vi "PICInit.vi"(2 "Error In":errorcluster, 3 "Enum":enum32{"9600", "115200"}(ring), 4 "VISA resource name":refnum<visa-resource-name>) -> (0 "error out":errorcluster, 1 "VISA resource name out":refnum<visa-resource-name>)   [LabVIEW 2012]
uses:
  <vilib>/Instr/_visa.llb/VISA Find Search Mode.ctl
  <vilib>/Instr/_visa.llb/VISA Configure Serial Port (Instr).vi
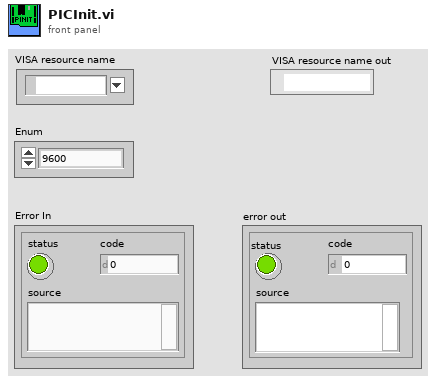
[diagram p1: front panel]
types:
  T1 = typedef "VISA Find Search Mode.ctl" = u32
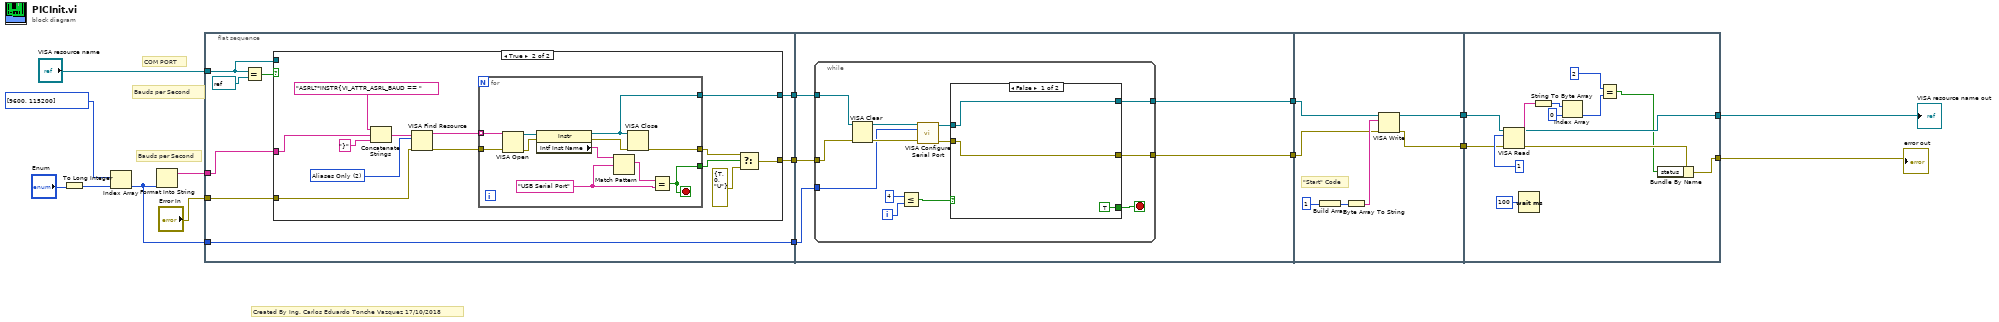
[diagram p0: block diagram]
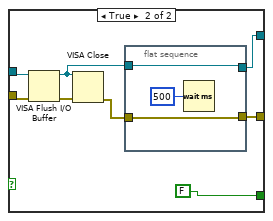
[diagram p3: hidden frame]
diagram:
  # "Created By Ing. Carlos Eduardo Tonche Vazquez 17/10/2018"
  # "COM PORT"
  # "Bauds per Second"
  # "Bauds per Second"
  n1 = To Long Integer(number="Enum") -> (32bit integer=w14:i32)
  n2 = Index Array(array=u32[] [9600, 115200], index=w14) -> (element=w11:u32)
  n3 = Format Into String(w11) -> (resulting string=w13:string)  [unwired: 3 in, 1 out]
  n4 = flat-sequence {
    tunnel: w13 -> [w22]
    tunnel: "VISA resource name" -> [w18]
    tunnel: w11 -> [w17]
    tunnel: "Error In" -> [w21]
    tunnel: [w20] -> w9
    tunnel: [w19] -> w8
    tunnel: [w17] -> w7
    tunnel: w9 -> [w55]
    tunnel: w8 -> [w54]
    tunnel: w7 -> [w53]
    tunnel: [w52] -> w6
    tunnel: [w51] -> w5
    tunnel: w6 -> [w86]
    tunnel: w5 -> [w85]
    tunnel: [w84] -> w2
    tunnel: [w83] -> w1
    tunnel: [w93] -> w3
    tunnel: [w92] -> w4
    tunnel: w2 -> [w95]
    tunnel: w1 -> [w94]
    frame #0 {
      n5 = Equal?(x=w18, y=refnum<visa-resource-name> refnum) -> (x = y?=w23:bool)
      n6 = case shown="True" w23 {
        tunnel: w22 -> [_ w37]
        tunnel: w21 -> [w25 w34]
        tunnel: [w25 w28] -> w20
        tunnel: [w26 w27] -> w19
        tunnel: w18 -> [w26 _]
        frame False {
        }
        frame True {
          w35 = T1 2 items=["Canonical Names Only"=0, "Aliases Only"=2, "Include Matching Aliases"=3, "Include All Aliases"=4] ("Search Mode")
          n7 = Concatenate Strings("ASRL?*INSTR{VI_ATTR_ASRL_BAUD == " ("string"), w37, "}" ("string")) -> (w36:string)
          n8 = VISA Find Resource(8:w34, 10:w35, 11:w36) -> (0:w33:errorcluster, 3:w32:string[])  [unwired: 1 out]
          n9 = for {
            tunnel: w33 -> [w50]
            tunnel: w32 -> [w49] mode=indexing
            tunnel: [w42] -> w27
            tunnel: [w41] -> w31
            tunnel: [w40] -> w30
            stop <- w41 stop-if-true
            w45 = "USB Serial Port"
            n10 = VISA Open(error in (no error)=w50, VISA resource name=w49) -> (VISA resource name=w47:refnum<visa-resource-name>, error out=w48:errorcluster)  [unwired: 3 in]
            n11 = property class="Instr"(reference=w47, error in=w48) -> (reference out=w42:refnum<visa-resource-name>, error out=w43:errorcluster, "Intf Inst Name"=w46:string)
            n12 = Match Pattern(string=w46, regular expression=w45) -> (match substring=w44:string)  [unwired: 1 in, 3 out]
            n13 = VISA Close(VISA resource name=w42, error in (no error)=w43) -> (error out=w40:errorcluster)
            n14 = Equal?(x=w44, y=w45) -> (x = y?=w41:bool)
          }
          n15 = Select(t=w30, s=w31, f=errorcluster {"status"=TRUE, "code"=0, "source"="U"}) -> (s? t:f=w28:errorcluster)
        }
      }
    }
    frame #1 {
      n16 = while {
        tunnel: w55 -> [w68]
        tunnel: w54 -> [w67]
        tunnel: w53 -> [w64]
        tunnel: [w57] -> w52
        tunnel: [w56] -> w51
        i -> [w63]
        stop <- w58 stop-if-true
        n17 = VISA Clear(VISA resource name=w67, error in (no error)=w68) -> (VISA resource name out=w66:refnum<visa-resource-name>, error out=w65:errorcluster)
        n18 = Less Or Equal?(x=4, y=w63) -> (x <= y?=w62:bool)
        n19 = call-poly "VISA Configure Serial Port"("VISA resource name"=w66, "baud rate (9600)"=w64, "error in (no error)"=w65) -> ("VISA resource name out"=w59:refnum<visa-resource-name>, "error out"=w60:errorcluster)  [unwired: 11 in]
        n20 = case shown="False" w62 {
          tunnel: w60 -> [w70 w78]
          tunnel: w59 -> [w71 w74]
          tunnel: [TRUE FALSE] -> w58
          tunnel: [w70 w75] -> w57
          tunnel: [w71 w72] -> w56
          frame False {
          }
          frame True {
            n21 = VISA Flush I/O Buffer(VISA resource name=w74, error in (no error)=w78) -> (VISA resource name out=w73:refnum<visa-resource-name>, error out=w79:errorcluster)  [unwired: 1 in]
            n22 = VISA Close(VISA resource name=w73, error in (no error)=w79) -> (error out=w76:errorcluster)
            n23 = flat-sequence {
              tunnel: [w81] -> w75
              tunnel: w76 -> [w81]
              tunnel: w73 -> [w80]
              tunnel: [w80] -> w72
              frame #0 {
                n24 = Wait (ms)(milliseconds to wait=u32 500) -> ()  [unwired: 1 out]
              }
            }
          }
        }
      }
    }
    frame #2 {
      # "\"Start\" Code"
      n25 = Build Array(u8 1) -> (w88:u8[])
      n26 = Byte Array To String(unsigned byte array=w88) -> (string=w87:string)
      n27 = VISA Write(VISA resource name=w85, write buffer=w87, error in (no error)=w86) -> (VISA resource name out=w83:refnum<visa-resource-name>, error out=w84:errorcluster)  [unwired: 1 out]
    }
    frame #3 {
      n28 = VISA Read(VISA resource name=w94, byte count=u32 1, error in (no error)=w95) -> (VISA resource name out=w93:refnum<visa-resource-name>, read buffer=w101:string, error out=w96:errorcluster)  [unwired: 1 out]
      n29 = Wait (ms)(milliseconds to wait=u32 100) -> ()  [unwired: 1 out]
      n30 = String To Byte Array(string=w101) -> (unsigned byte array=w100:u8[])
      n31 = Index Array(array=w100, index=0) -> (element=w98:u8)
      n32 = Equal?(x=u8 2, y=w98) -> (x = y?=w90:bool)
      n33 = Bundle By Name(cluster=w96, "status"=w90) -> (w92:errorcluster)
    }
  }
  "error out" <- w4
  "VISA resource name out" <- w3
